vi "测量流程.vi"(11 "控制命令":T1(ring)) -> ()   [LabVIEW 2016, in "斯坦道氨氮.lvlib"]
panel:
  out "x-y":dbl
  out "当前时间":timestamp
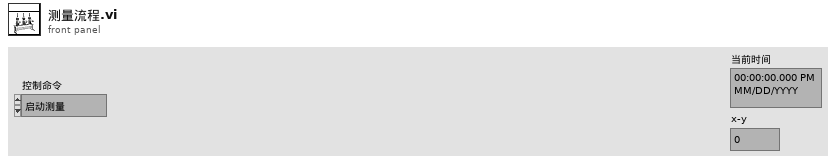
[diagram p1: front panel]
types:
  T1 = enum16{"启动测量", "标样核查", "零点核查", "跨度核查", "空白测试", "平行样测试", "加标回收", "空白校准", "标样校准", "初始化（清洗）", "停止测试", "仪器重启", "校时", "模式设置", "测量间隔设置"}
  T2 = cluster{"站号":u16, "量程切换":enum32{"H", "L", "AUTO"}, "控制命令":enum16{"启动测量", "标样核查", "零点核查", "跨度核查", "空白测试", "平行样测试", "加标回收", "空白校准", "标样校准", "初始化（清洗）", "停止测试", "仪器重启", "校时", "模式设置", "测量间隔设置"}, "模式设置":enum16{"待机", "连续模式", "周期模式", "定点模式", "受控模式", "手动模式"}, "测量间隔":u16}
  T3 = cluster{"时间标识":timestamp, "设备":string, "日志信息":string, "流程参数":string}
  T4 = enum16{"空闲", "水样测试", "标样核查", "零点核查", "跨度核查", "空白测试", "平行样测试", "加标回收", "空白校准", "标样校准", "初始化（清洗）"}
  T5 = cluster{"系统时间":timestamp, "工作状态":u16, "测量模式":enum16{"待机", "连续模式", "周期模式", "定点模式", "受控模式", "手动模式"}, "告警代码":u16, "故障代码":u16, "日志代码":u16, "软件版本":u16, "F0":sgl, "F1":sgl, "F2":sgl, "F3":sgl, "T":sgl, "H":sgl, "id":u16, "flowid":u16, "量程":u16, "总磷控温温度1":sgl, "营养盐控温温度2":sgl, "ADC":sgl}
  T6 = cluster{"水样测试量程模式":enum16{"H", "L", "AUTO"}, "空白核查量程模式":enum16{"H", "L", "AUTO"}, "跨度核查量程模式":enum16{"H", "L", "AUTO"}, "加标回收量程模式":enum16{"H", "L", "AUTO"}, "标样核查量程模式":enum16{"H", "L", "AUTO"}}
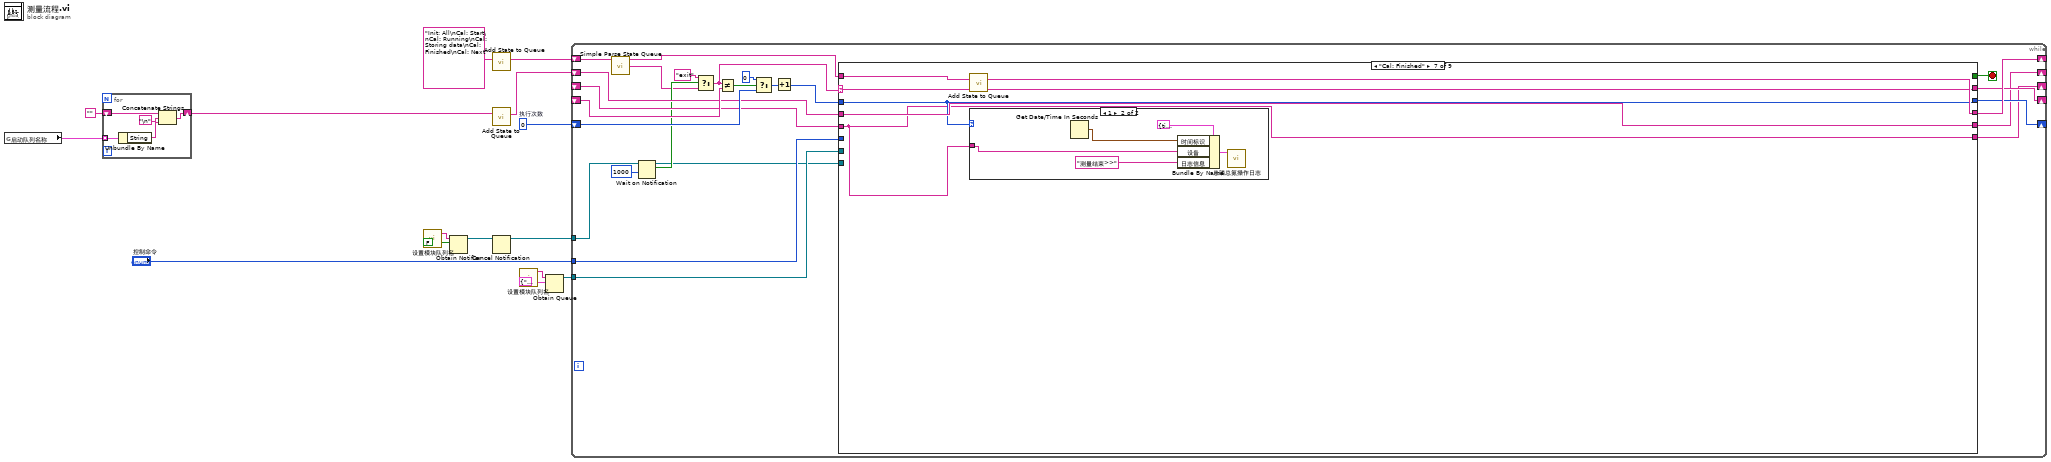
[diagram p0: block diagram]
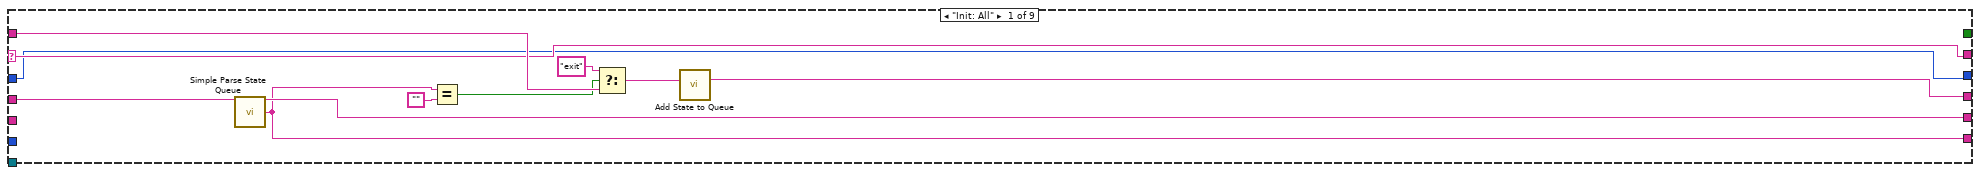
[diagram p2: hidden frame]
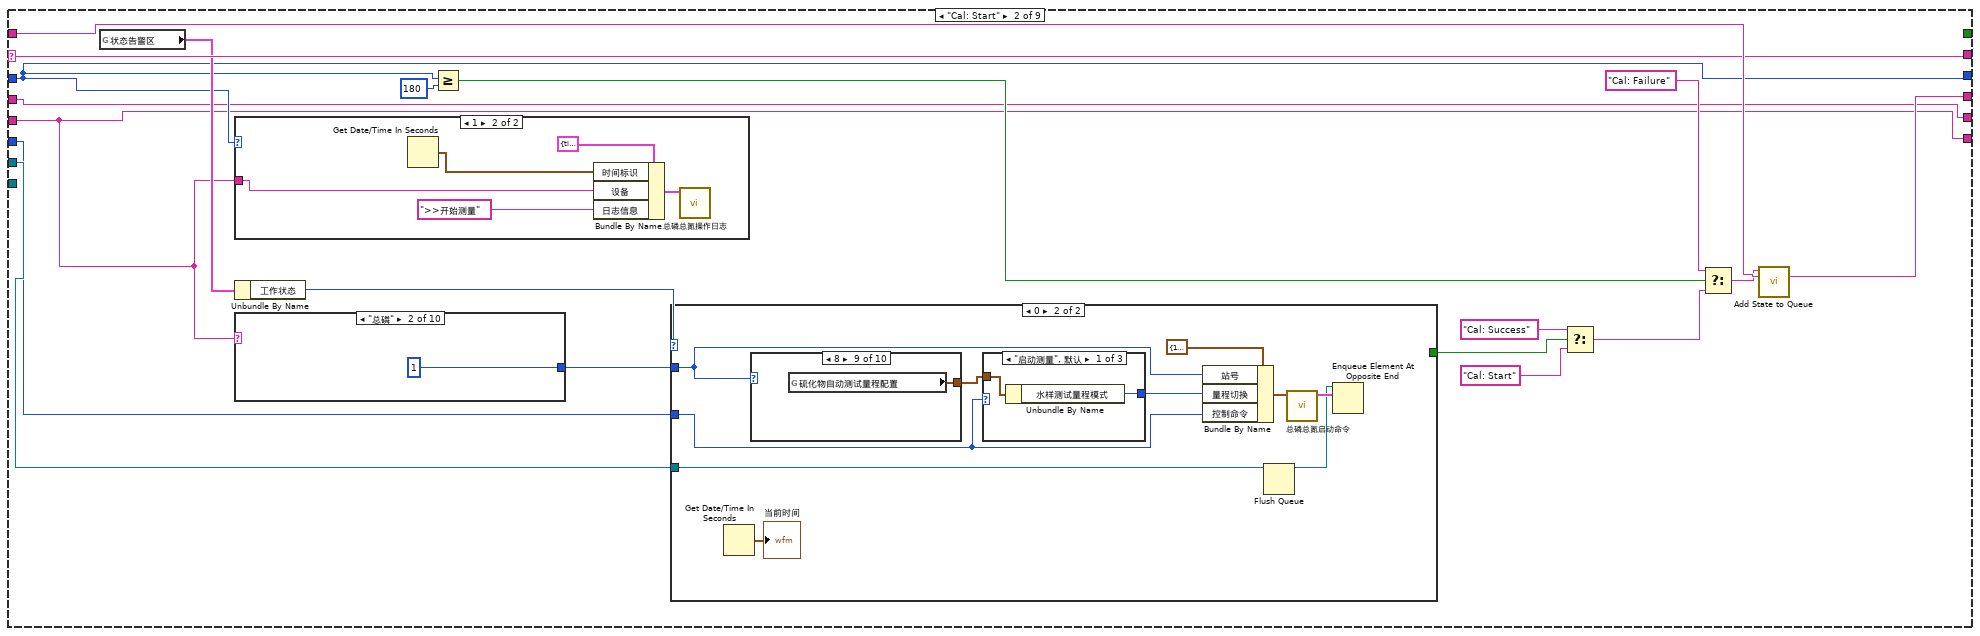
[diagram p3: hidden frame]
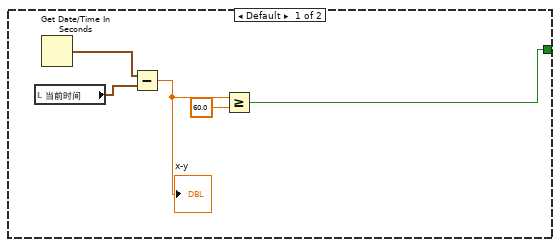
[diagram p4: hidden frame]
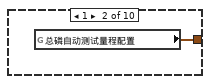
[diagram p6: hidden frame]
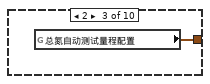
[diagram p7: hidden frame]
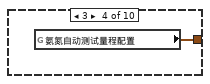
[diagram p8: hidden frame]
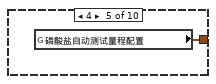
[diagram p9: hidden frame]
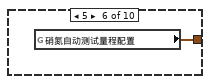
[diagram p10: hidden frame]
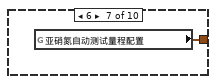
[diagram p11: hidden frame]
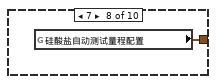
[diagram p12: hidden frame]
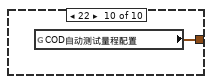
[diagram p13: hidden frame]
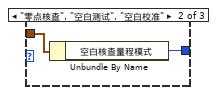
[diagram p14: hidden frame]
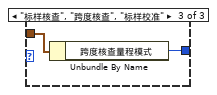
[diagram p15: hidden frame]
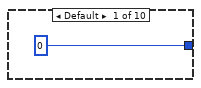
[diagram p16: hidden frame]
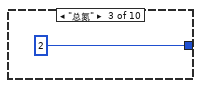
[diagram p17: hidden frame]
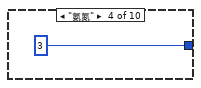
[diagram p18: hidden frame]
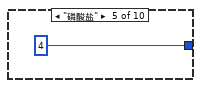
[diagram p19: hidden frame]
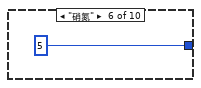
[diagram p20: hidden frame]
diagram:
  w9 = 0  # 执行次数
  n1 = global read "总磷总氮断电保存全局变量.vi" "启动队列名称"() -> (w1:cluster{"String":string, "Value":u16}[])
  n2 = for {
    shift-right: [w19] -> w2
    shift-left: "" -> [w20]
    tunnel: w1 -> [w18] mode=indexing
    n3 = Unbundle By Name(w18) -> ("String"=w17:string)
    n4 = Concatenate Strings(w20, "\n", w17) -> (w19:string)
  }
  n5 = call "设置模块队列名.vi"() -> ("Msg"=w6:string)  [unwired: 5 in]
  n6 = Obtain Notifier(name (unnamed)=w6, notification data type=FALSE) -> (notifier out=w14:refnum<notifier>)  [unwired: 2 in, 2 out]
  n7 = call "Add State to Queue.vi"("State(s) In (\"\")"="Init: All\nCal: Start\nCal: Running\nCal: Storing data\nCal: Finished\nCal: Next" ("State(s) In (\"\")")) -> ("States Out"=w12:string)  [unwired: 14 in]
  n8 = call "Add State to Queue.vi"("State(s) In (\"\")"=w2) -> ("States Out"=w7:string)  [unwired: 14 in]
  n9 = Cancel Notification(0:w14) -> (8:w4:refnum<notifier>)  [unwired: 1 in, 2 out]
  n10 = call "设置模块队列名.vi"() -> ("Msg"=w5:string)  [unwired: 5 in]
  n11 = Obtain Queue(name (unnamed)=w5, element data type=cluster{"命令":string, "data":variant} {"命令"="", "data"=variant}) -> (queue out=w10:refnum<queue>)  [unwired: 3 in, 2 out]
  n12 = while {
    tunnel: w10 -> [w43]
    shift-right: [w42] -> _
    shift-left: w12 -> [w45]
    shift-right: [w35] -> _
    shift-left: w9 -> [w38]
    shift-right: [w41] -> _
    shift-left: _ -> [w40]
    tunnel: "控制命令" -> [w33]
    shift-right: [w29] -> _
    shift-left: w7 -> [w31]
    shift-right: [w30] -> _
    shift-left: _ -> [w28]
    tunnel: w4 -> [w26]
    stop <- w32 stop-if-true
    n13 = call "Simple Parse State Queue.vi"("State Queue"=w45) -> ("Remain States"=w44:string, "Next State"=w23:string)  [unwired: 13 in]
    n14 = Wait on Notification(notifier=w26, timeout in ms (-1)=1000 ("超时毫秒(-1)")) -> (notifier out=w21:refnum<notifier>, notification=w25:bool)  [unwired: 2 in, 2 out]
    n15 = Select(t="exit", s=w25, f=w23) -> (s? t:f=w22:string)
    n16 = Not Equal?(x=w22, y=w40) -> (x != y?=w39:bool)
    n17 = Select(t=0, s=w39, f=w38) -> (s? t:f=w36:i32)
    n18 = Increment(x=w36) -> (x+1=w34:i32)
    n19 = case shown="\"Cal: Finished\"" w22 {
      selector: w22 -> [w52 w73 w124 w139 w145 w159 w175 w186 w193]
      tunnel: w44 -> [w54 w75 w126 _ w156 w164 w177 _ w194]
      tunnel: w43 -> [_ w71 _ _ _ _ _ _ w189]
      tunnel: [w56 w74 w125 w140 w155 w163 w176 "Init: All\nCal: Start\nCal: Running\nCal: Storing data\nCal: Finished\nCal: Next" ("State(s) In (\"\")") w194] -> w42
      tunnel: [w52 w73 w124 w139 w145 w159 w175 w186 w193] -> w41
      tunnel: [w51 w68 w123 w138 w148 w162 w173 w185 w192] -> w35
      tunnel: w34 -> [w51 w68 w123 w138 w148 w162 w173 w185 w192]
      tunnel: w33 -> [_ w70 _ _ _ _ _ _ _]
      tunnel: [_ _ _ _ _ _ _ _ TRUE] -> w32
      tunnel: w31 -> [w50 w57 w122 w132 w142 w166 w174 w184 w191]
      tunnel: [w48 w58 w121 w131 w141 w165 w172 w183 w190] -> w30
      tunnel: [w49 w57 w122 w132 w142 w166 w174 w184 w191] -> w29
      tunnel: w28 -> [_ w58 w121 w131 w141 w165 w172 w183 w190]
      tunnel: w21 -> [_ _ _ _ _ _ _ _ w188]
      frame "Init: All" {
        n20 = call "Simple Parse State Queue.vi"("State Queue"=w50) -> ("Remain States"=w49:string, "Next State"=w48:string)  [unwired: 13 in]
        n21 = Equal?(x=w48, y="") -> (x = y?=w46:bool)
        n22 = Select(t="exit", s=w46, f=w54) -> (s? t:f=w53:string)
        n23 = call "Add State to Queue.vi"("State(s) In (\"\")"=w53) -> ("States Out"=w56:string)  [unwired: 14 in]
      }
      frame "Cal: Start" {
        n24 = global read "VAR总磷总氮全局变量.vi" "状态告警区"() -> (w72:T5)
        n25 = case shown="1" w68 {
          tunnel: w58 -> [_ w116]
          frame 0, Default {
          }
          frame 1 {
            n26 = Get Date/Time In Seconds() -> (seconds since 1Jan1904=w120:timestamp)
            n27 = Bundle By Name(cluster=T3 {"时间标识"=timestamp(0 s since 1904-01-01), "设备"="", "日志信息"="", "流程参数"=""} ("data in"), "时间标识"=w120, "设备"=w116, "日志信息"=">>开始测量") -> (w119:T3)
            n28 = call "总磷总氮操作日志.vi"("data in"=w119) -> ()  [unwired: 11 in]
          }
        }
        n29 = Unbundle By Name(w72) -> ("工作状态"=w59:u16)
        n30 = case shown="\"总磷\"" w58 {
          tunnel: [0 1 2 3 4 5 6 7 8 22] -> w69
          frame Default {
          }
          frame "总磷" {
          }
          frame "总氮" {
          }
          frame "氨氮" {
          }
          frame "磷酸盐" {
          }
          frame "硝氮" {
          }
          frame "亚硝氮" {
          }
          frame "硅酸盐" {
          }
          frame "硫化物" {
          }
          frame "COD" {
          }
        }
        n31 = Greater Or Equal?(x=w68, y=180) -> (x >= y?=w66:bool)
        n32 = case shown="0" w59 {
          tunnel: w70 -> [_ w86]
          tunnel: w71 -> [_ w89]
          tunnel: [w76 _] -> w63
          tunnel: w69 -> [_ w84]
          frame Default {
            n33 = local read "当前时间"() -> (w80:timestamp)
            n34 = Get Date/Time In Seconds() -> (seconds since 1Jan1904=w79:timestamp)
            n35 = Subtract(x=w79, y=w80) -> (x-y=w78:dbl)
            "x-y" <- w78
            n36 = Greater Or Equal?(x=w78, y=60.0) -> (x >= y?=w76:bool)
          }
          frame 0 {
            n37 = Get Date/Time In Seconds() -> (seconds since 1Jan1904=→"当前时间":timestamp)
            n38 = case shown="8" w84 {
              tunnel: [_ w91 w92 w93 w94 w95 w96 w97 w98 w99] -> w85
              frame 0, Default {
              }
              frame 1 {
                n39 = global read "总磷总氮断电保存全局变量.vi" "总磷自动测试量程配置"() -> (w91:T6)
              }
              frame 2 {
                n40 = global read "总磷总氮断电保存全局变量.vi" "总氮自动测试量程配置"() -> (w92:T6)
              }
              frame 3 {
                n41 = global read "总磷总氮断电保存全局变量.vi" "氨氮自动测试量程配置"() -> (w93:T6)
              }
              frame 4 {
                n42 = global read "总磷总氮断电保存全局变量.vi" "磷酸盐自动测试量程配置"() -> (w94:T6)
              }
              frame 5 {
                n43 = global read "总磷总氮断电保存全局变量.vi" "硝氮自动测试量程配置"() -> (w95:T6)
              }
              frame 6 {
                n44 = global read "总磷总氮断电保存全局变量.vi" "亚硝氮自动测试量程配置"() -> (w96:T6)
              }
              frame 7 {
                n45 = global read "总磷总氮断电保存全局变量.vi" "硅酸盐自动测试量程配置"() -> (w97:T6)
              }
              frame 8 {
                n46 = global read "总磷总氮断电保存全局变量.vi" "硫化物自动测试量程配置"() -> (w98:T6)
              }
              frame 22 {
                n47 = global read "总磷总氮断电保存全局变量.vi" "COD自动测试量程配置"() -> (w99:T6)
              }
            }
            n48 = case shown="\"启动测量\", 默认" w86 {
              tunnel: w85 -> [w101 w103 w105]
              tunnel: [w100 w102 w104] -> w90
              frame "启动测量", Default {
                n49 = Unbundle By Name(w101) -> ("水样测试量程模式"=w100:enum16{"H", "L", "AUTO"})
              }
              frame "零点核查", "空白测试", "空白校准" {
                n50 = Unbundle By Name(w103) -> ("空白核查量程模式"=w102:enum16{"H", "L", "AUTO"})
              }
              frame "标样核查", "跨度核查", "标样校准" {
                n51 = Unbundle By Name(w105) -> ("跨度核查量程模式"=w104:enum16{"H", "L", "AUTO"})
              }
            }
            n52 = Bundle By Name(cluster=T2 {"站号"=1, "量程切换"=enum."AUTO", "控制命令"=enum."启动测量", "模式设置"=enum."待机", "测量间隔"=0} ("参数"), "站号"=w84, "量程切换"=w90, "控制命令"=w86) -> (w87:T2)
            n53 = Flush Queue(queue=w89) -> (queue out=w82:refnum<queue>)  [unwired: 1 in, 2 out]
            n54 = call "总磷总氮启动命令.vi"("参数"=w87) -> ("启动命令"=w83:cluster{"命令":string, "data":variant})  [unwired: 10 in]
            n55 = Enqueue Element At Opposite End(queue=w82, element=w83) -> ()  [unwired: 2 in, 3 out]
          }
        }
        n56 = Select(t="Cal: Success" ("State(s) In (\"\")"), s=w63, f="Cal: Start" ("State(s) In (\"\")")) -> (s? t:f=w61:string)
        n57 = Select(t="Cal: Failure" ("State(s) In (\"\")"), s=w66, f=w61) -> (s? t:f=w64:string)
        n58 = call "Add State to Queue.vi"("State(s) In Front (\"\")"=w64, "State(s) In (\"\")"=w75) -> ("States Out"=w74:string)  [unwired: 13 in]
      }
      frame "Cal: Success" {
        n59 = Get Date/Time In Seconds() -> (seconds since 1Jan1904=w129:timestamp)
        n60 = Bundle By Name(cluster=T3 {"时间标识"=timestamp(0 s since 1904-01-01), "设备"="", "日志信息"="", "流程参数"=""} ("data in"), "时间标识"=w129, "设备"=w121, "日志信息"="-->>启动成功") -> (w128:T3)
        n61 = call "总磷总氮操作日志.vi"("data in"=w128) -> ()  [unwired: 11 in]
        n62 = call "Add State to Queue.vi"("State(s) In (\"\")"=w126) -> ("States Out"=w125:string)  [unwired: 14 in]
      }
      frame "Cal: Failure" {
        n63 = Get Date/Time In Seconds() -> (seconds since 1Jan1904=w136:timestamp)
        n64 = Bundle By Name(cluster=T3 {"时间标识"=timestamp(0 s since 1904-01-01), "设备"="", "日志信息"="", "流程参数"=""} ("data in"), "时间标识"=w136, "设备"=w131, "日志信息"="-->>启动失败") -> (w135:T3)
        n65 = call "总磷总氮操作日志.vi"("data in"=w135) -> ()  [unwired: 11 in]
        n66 = call "Add State to Queue.vi"("State(s) In (\"\")"="exit" ("State(s) In (\"\")")) -> ("States Out"=w140:string)  [unwired: 14 in]
      }
      frame "Cal: Running" {
        n67 = global read "VAR总磷总氮全局变量.vi" "状态告警区"() -> (w152:T5)
        n68 = Unbundle By Name(w152) -> ("工作状态"=w153:u16)
        n69 = Less Or Equal?(x=w148, y=7200) -> (x <= y?=w146:bool)
        n70 = Select(t=w145, s=w146, f="exit") -> (s? t:f=w144:string)
        n71 = Equal?(x=w153, y=T4."空闲") -> (x = y?=w151:bool)
        n72 = Select(t="", s=w151, f=w144) -> (s? t:f=w149:string)
        n73 = call "Add State to Queue.vi"("State(s) In Front (\"\")"=w149, "State(s) In (\"\")"=w156) -> ("States Out"=w155:string)  [unwired: 13 in]
      }
      frame "Cal: Storing data" {
        n74 = case shown="1" w162 {
          tunnel: w165 -> [_ w167]
          frame 0, Default {
          }
          frame 1 {
            n75 = Get Date/Time In Seconds() -> (seconds since 1Jan1904=w171:timestamp)
            n76 = Bundle By Name(cluster=T3 {"时间标识"=timestamp(0 s since 1904-01-01), "设备"="", "日志信息"="", "流程参数"=""} ("data in"), "时间标识"=w171, "设备"=w167, "日志信息"="-->>存储数据") -> (w170:T3)
            n77 = call "总磷总氮操作日志.vi"("data in"=w170) -> ()  [unwired: 11 in]
          }
        }
        n78 = Less Or Equal?(x=w162, y=10) -> (x <= y?=w160:bool)
        n79 = Select(t=w159, s=w160, f="") -> (s? t:f=w157:string)
        n80 = call "Add State to Queue.vi"("State(s) In Front (\"\")"=w157, "State(s) In (\"\")"=w164) -> ("States Out"=w163:string)  [unwired: 13 in]
      }
      frame "Cal: Finished" {
        n81 = call "Add State to Queue.vi"("State(s) In (\"\")"=w177) -> ("States Out"=w176:string)  [unwired: 14 in]
        n82 = case shown="1" w173 {
          tunnel: w172 -> [_ w178]
          frame 0, Default {
          }
          frame 1 {
            n83 = Get Date/Time In Seconds() -> (seconds since 1Jan1904=w182:timestamp)
            n84 = Bundle By Name(cluster=T3 {"时间标识"=timestamp(0 s since 1904-01-01), "设备"="", "日志信息"="", "流程参数"=""} ("data in"), "时间标识"=w182, "设备"=w178, "日志信息"="测量结束>>") -> (w181:T3)
            n85 = call "总磷总氮操作日志.vi"("data in"=w181) -> ()  [unwired: 11 in]
          }
        }
      }
      frame "Cal: Next" {
      }
      frame "exit", Default {
        n86 = Release Queue(queue=w189) -> ()  [unwired: 2 in, 3 out]
        n87 = Release Notifier(notifier=w188) -> ()  [unwired: 2 in, 3 out]
      }
    }
  }
